vi "line to strings.vi"(11 "line":T1) -> (3 "strings":string[](array[string]))   [LabVIEW 2013, in "EthernetIP editor node.lvclass"]
uses:
  EthernetIP editor node.lvclass
  table line.ctl
  channel/EthernetIP Channel.lvclass
  <vilib>/NI/Tag Bus/tag/tag descriptor.lvclass/tag descriptor.ctl
  channel/EthernetIP Channel.lvclass/EthernetIP Channel.ctl
  <vilib>/NI/Tag Bus Module Framework/channel/TBM channel.lvclass/TBM channel.ctl
  <vilib>/NI/Tag Bus/tag/read tag name.vi
  channel/Read Instance ID.vi
  <vilib>/NI/Tag Bus Module Framework/channel/Read channel classification.vi
  channel/Read byte index.vi
  <vilib>/NI/Tag Bus/tag/read data type.vi
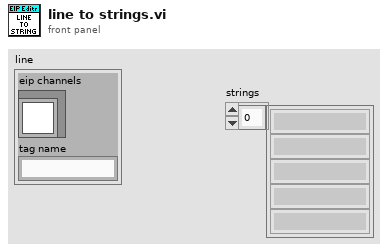
[diagram p1: front panel]
types:
  T1 = typedef "EthernetIP editor node.lvclass/table line.ctl" = cluster{"eip channels":refnum<class "EthernetIP Channel.lvclass">, "tag name":string}
  T2 = typedef "TBM channel.lvclass/channel classification.ctl" = enum16{"input data", "output data", "processing parameter", "processing result"}
  T3 = typedef "tag bus.lvlib/tag descriptor.lvclass/Data Type.ctl" = enum16{"Double", "Single", "I64", "I32", "I16", "I8", "U64", "U32", "U16", "U8", "Boolean", "String", "Array of Double", "Array of Single", "Array of I64", "Array of I32", "Array of I16", "Array of I8", "Array of U64", "Array of U32", "Array of U16", "Array of U8", "Array of Boolean", "Array of String"}
  T4 = typedef "EthernetIP configuration.lvclass/assembly type.ctl" = enum32{"Producing", "Consuming"}
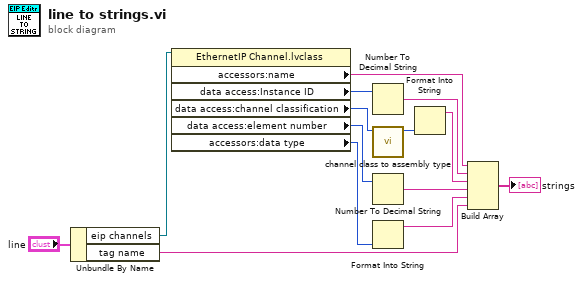
[diagram p0: block diagram]
diagram:
  n1 = Unbundle By Name("line") -> ("eip channels"=w9:refnum<class "EthernetIP Channel.lvclass">, "tag name"=w12:string)
  n2 = property class="EthernetIP Channel.lvclass"(reference=w9) -> ("accessors:name"=w7:string, "data access:Instance ID"=w4:u32, "data access:channel classification"=w6:T2, "data access:element number"=w2:i32, "accessors:data type"=w8:T3)  [unwired: 1 in, 2 out]
  n3 = Number To Decimal String(number=w4) -> (decimal integer string=w3:string)  [unwired: 1 in]
  n4 = call "channel class to assembly type.vi"("channel classification"=w6) -> ("assembly types"=w5:T4)  [unwired: 10 in]
  n5 = Number To Decimal String(number=w2) -> (decimal integer string=w1:string)  [unwired: 1 in]
  n6 = Format Into String(w8) -> (resulting string=w13:string)  [unwired: 3 in, 1 out]
  n7 = Format Into String(w5) -> (resulting string=w10:string)  [unwired: 3 in, 1 out]
  n8 = Build Array(w7, w3, w10, w1, w13, w12) -> (→"strings":string[])
